vi "sensor tester.vi"   [LabVIEW 2012, in "Omni2013.lvrbt"]
uses:
  Omni2013.lvrbt
  <vilib>/NXT/Block Support/NXT_InputPort.ctl
  <vilib>/NXT/HiTechnic/HiTechnic Config/HiTechnic IRSeeker Mode1200Hz.vi
  <vilib>/NXT/HiTechnic/HiTechnic Read/HiTechnic IRSeeker Sensor_AC all.vi
  <vilib>/NXT/Dual Mode Library/Display/drawNumber.vi
  <vilib>/NXT/Dual Mode Library/Sensors/Sonar_cm.vi
types:
  T1 = typedef "NXT_InputPort.ctl" = u8
  T2 = typedef "LVHSConnector.ctl" = refnum<class "BrickReference.lvclass">
  T3 = cluster{"Direction (0-9)":i16, "Signal Strength (Array)":u8[]}
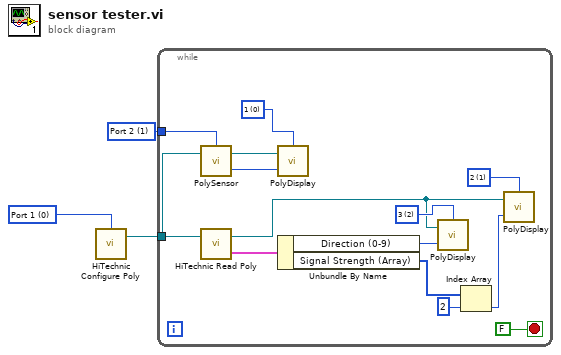
[diagram p0: block diagram]
diagram:
  w1 = T1 1 items=["Port 1", "Port 2", "Port 3", "Port 4"] ("Port (Port 4)")
  w3 = T1 0 items=["Port 1", "Port 2", "Port 3", "Port 4"] ("Port")
  n1 = call-poly <vilib>:"HiTechnic Configure Poly.vi"("Port"=w3) -> ("NXT"=w2:T2)  [unwired: 3 in]
  n2 = while {
    tunnel: w2 -> [w17]
    tunnel: w1 -> [w14]
    stop <- FALSE stop-if-true
    w6 = i16 2 items=["1", "2", "3", "4", "5", "6", "7", "8"] ("Line")
    w12 = i16 1 items=["1", "2", "3", "4", "5", "6", "7", "8"] ("Line")
    w13 = i16 0 items=["1", "2", "3", "4", "5", "6", "7", "8"] ("Line")
    n3 = call-poly <vilib>:"PolySensor.vi"("NXT"=w17, "Port (Port 4)"=w14) -> ("Distance (cm)"=w16:i16, "NXT"=w15:T2)  [unwired: 1 in]
    n4 = call-poly <vilib>:"HiTechnic Read Poly.vi"("NXT"=w17) -> ("All Info"=w11:T3, "NXT"=w5:T2)  [unwired: 2 in]
    n5 = call-poly <vilib>:"PolyDisplay.vi"("number"=w16, "NXT"=w15, "Line"=w13) -> ()  [unwired: 1 in, 1 out]
    n6 = Unbundle By Name(w11) -> ("Direction (0-9)"=w7:i16, "Signal Strength (Array)"=w10:u8[])
    n7 = call-poly <vilib>:"PolyDisplay.vi"("number"=w7, "NXT"=w5, "Line"=w6) -> ()  [unwired: 1 in, 1 out]
    n8 = Index Array(array=w10, index=2) -> (element=w8:u8)
    n9 = call-poly <vilib>:"PolyDisplay.vi"("number"=w8, "NXT"=w5, "Line"=w12) -> ()  [unwired: 1 in, 1 out]
  }
